vi "HB_ThreadPool.MainDIMEventListenerTask.vi"() -> ()   [LabVIEW 2009, in "HB_DIM_Examples.lvlib"]
doc: "Simple application to test the HGF_ThreadPool with a simple class."
uses:
  HB_DIM_Examples.lvlib
  HB_Factory/HB_Factory.lvclass
  lib.lib/HGF_LVC/HGF_BaseClasses/HGF_Factory/HGF_Factory.lvclass
  lib.lib/HGF_LVC/HGF_BaseClasses/HGF_Event/HGF_Event.lvclass
  lib.lib/HGF_LVC/HGF_BaseClasses/HGF_ThreadTask/HGF_ThreadTask.lvclass
  HB_Simple/HB_Simple.lvclass
  lib.lib/HGF_LVC/HGF_BaseClasses/HGF_NetworkVisitor/HGF_NetworkVisitor.lvclass
  lib.lib/HGF_LVC/HGF_BaseClasses/HGF_TriggeredEvent/HGF_TriggeredEvent.lvclass
  lib.lib/HGF_LVC/HGF_BaseClasses/HGF_PVSubscriber/HGF_PVSubscriber.lvclass
  lib.lib/HGF_LVC/HGF_DIM/HGF_DIMFactory/HGF_DIMFactory.lvclass/HGF_DIMFactory.lvclass
  lib.lib/HGF_LVC/HGF_ObjectManager/HGF_OMFactory/HGF_OMFactory.lvclass
  lib.lib/HGF_LVC/HGF_DIM/HGF_DIMDataConverter/HGF_DIMDataConverter.lvclass
  lib.lib/HGF_LVC/HGF_DIM/HGF_DIMService/HGF_DIMService.lvclass
  lib.lib/HGF_LVC/HGF_BaseClasses/HGF_ThreadPool/HGF_ThreadPool.lvclass
  lib.lib/HGF_LVC/HGF_BaseClasses/HGF_Reference/HGF_Reference.lvclass
  lib.lib/HGF_LVC/HGF_Auxiliary/HGF_Auxiliary.lvlib
  lib.lib/HGF_LVC/HGF_ObjectManager/HGF_ObjectManager.lvlib
  lib.lib/HGF_LVC/HGF_BaseClasses/HGF_Visitor/HGF_Visitor.lvclass
  lib.lib/HGF_LVC/HGF_BaseClasses/HGF_NetworkEvent/HGF_NetworkEvent.lvclass/HGF_NetworkEvent.lvclass
  lib.lib/HGF_LVC/HGF_DIM/HGF_DIMCommand/HGF_DIMCommand.lvclass
  lib.lib/DimLVEvent/LVDimInterface/LVDimInterface.lvlib
  lib.lib/HGF_LVC/HGF_DIM/HGF_DIMSubscriber/HGF_DIMSubscriber.lvclass
  lib.lib/HGF_LVC/HGF_BaseClasses/HGF_PVBase/HGF_PVBase.lvclass
panel:
  in  "y":dbl=1.0
  in  "Increment":bool
  out "objectName":string
  in  "nofObjects":i32=10
  out "Waveform Chart":dbl(graph)
  in  "timeout in ms (-1)":i32=3000
  out "nofTasksInQueueOut":i32
  out "nofTasksWaiting":i32
  out "autoIncrementLimit":i32=-1
  out "nofThreads":i32
  out "Default Destination timed out?":bool
  out "got object?":bool
  out "error":errorcluster
  in  "stop":bool
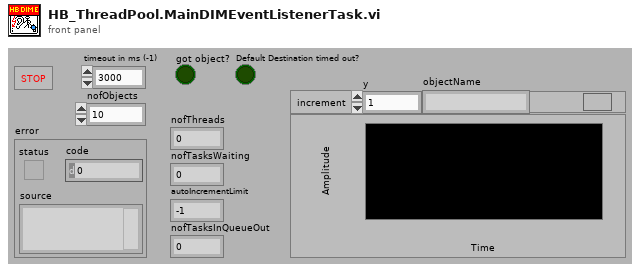
[diagram p1: front panel]
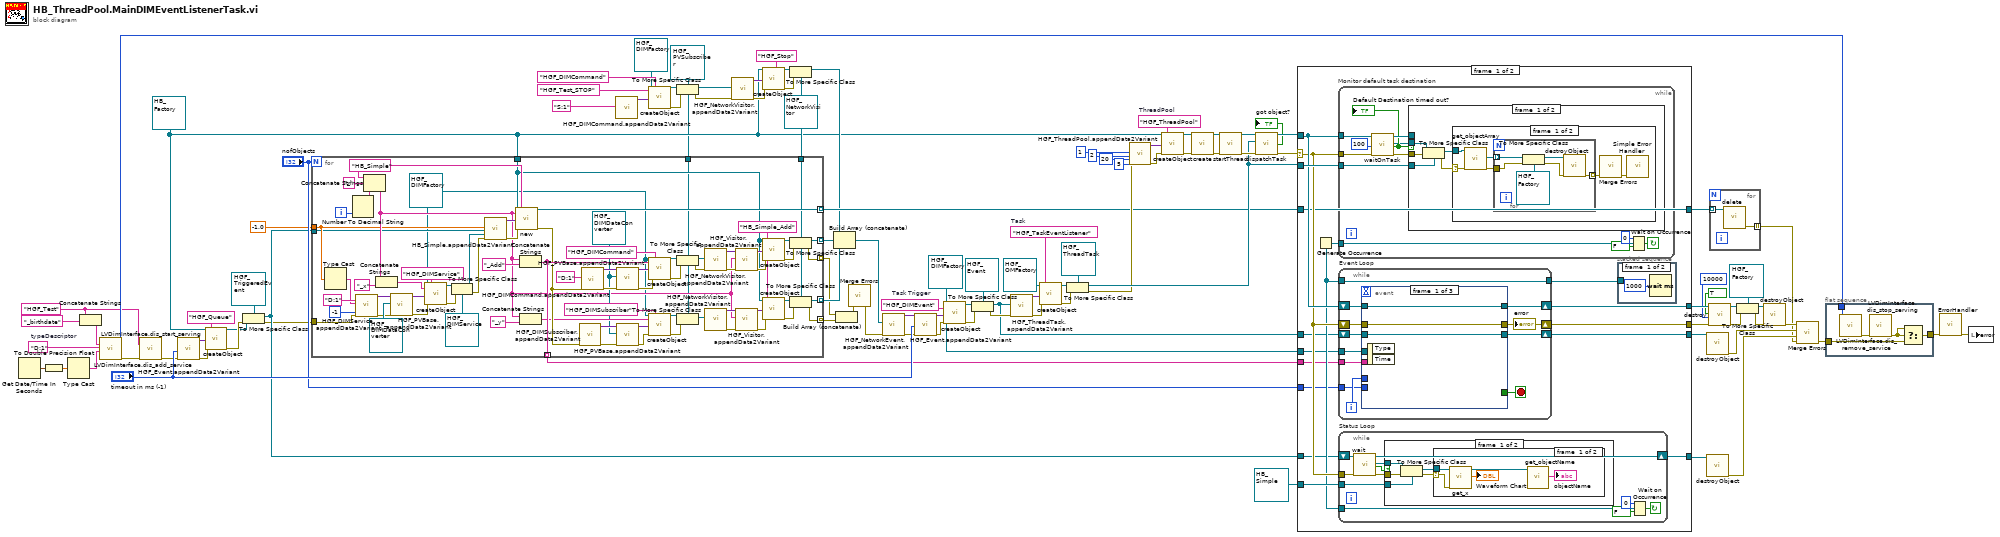
[diagram p0: block diagram]
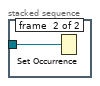
[diagram p2: hidden frame]
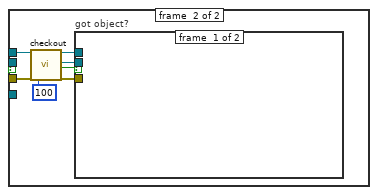
[diagram p6: hidden frame]
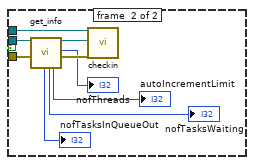
[diagram p7: hidden frame]
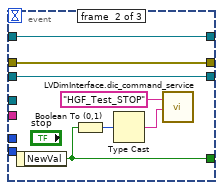
[diagram p8: hidden frame]
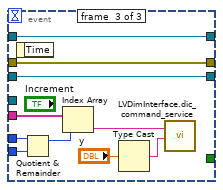
[diagram p9: hidden frame]
diagram:
  w2 = refnum<class "HGF_DIMFactory.lvclass"> refnum ("HGF_DIM.lvlib:HGF_DIMFactory.lvclass")
  w4 = refnum<class "HGF_PVSubscriber.lvclass"> refnum ("HGF_PVSubscriber")
  w7 = "HGF_Test" ("serverName")
  w13 = "D:1"  # typeDescriptor
  w35 = refnum<class "HGF_NetworkVisitor.lvclass"> refnum ("HGF_BaseClasses.lvlib:HGF_NetworkData.lvclass")
  w86 = "HGF_DIMEvent"  # Task Trigger
  w85 = "HGF_TaskEventListener"  # Task
  w78 = "HGF_ThreadPool"  # ThreadPool
  w19 = refnum<class "HB_Factory.lvclass"> refnum ("HB_Factory.lvclass")
  n1 = Get Date/Time In Seconds() -> (seconds since 1Jan1904=w10:timestamp)
  n2 = To Double Precision Float(number=w10) -> (double precision float=w11:dbl)
  n3 = Type Cast(x=w11) -> (*(type *) &x=w14:string)  [unwired: 1 out]
  n4 = Concatenate Strings(w7, "_birthdate") -> (w6:string)
  n5 = call "LVDimInterface.dis_add_service.vi"("serviceName"=w6, "typeDescriptor"=w13, "data"=w14) -> ("my_serviceID"=w9:i32, "error out"=w15:errorcluster)  [unwired: 2 in, 13 out]
  n6 = call "LVDimInterface.dis_start_serving.vi"("serverName"=w7, "error in (no error)"=w15) -> ("error out"=w12:errorcluster)  [unwired: 17 out]
  n7 = call "HGF_Event.appendData2Variant.vi"("timeout in ms (-1)"="timeout in ms (-1)", "error in (no error)"=w12) -> ("dup initData"=w64:variant, "error out"=w65:errorcluster)  [unwired: 1 in, 15 out]
  n8 = call "createObject.vi"("HGF_Factory"=w19, "initializationData"=w64, "error in (no error)"=w65, "className"="HGF_Queue") -> ("HGF_Object"=w61:refnum<class "HGF_Factory.lvclass">, "error out"=w62:errorcluster)  [unwired: 2 in, 12 out]
  n9 = To More Specific Class(target class=refnum<class "HGF_TriggeredEvent.lvclass"> refnum ("HGF_BaseClasses.lvlib:HGF_TriggeredEvent.lvclass"), reference=w61, error in=w62) -> (specific class reference=w18:refnum<class "HGF_TriggeredEvent.lvclass">, error out=w16:errorcluster)
  n10 = for {
    N: "nofObjects" -> [_]
    tunnel: [w173] -> w54 mode=indexing
    tunnel: w19 -> [w122]
    tunnel: [w163] -> w22 mode=indexing
    tunnel: [w156] -> w51 mode=indexing
    tunnel: [w162] -> w46 mode=indexing
    tunnel: w35 -> [w145]
    tunnel: [w144] -> w24 mode=indexing
    tunnel: [w143] -> w23 mode=indexing
    tunnel: w18 -> [w108]
    tunnel: -1.0 ("x") -> [w115]
    tunnel: w16 -> [w111]
    tunnel: w4 -> [w106]
    i -> [w175]
    w105 = refnum<class "HGF_DIMFactory.lvclass"> refnum ("HGF_DIM.lvlib:HGF_DIMFactory.lvclass")
    w130 = refnum<class "HGF_DIMDataConverter.lvclass"> refnum ("HGF_DIM.lvlib:HGF_DIMBaseType.lvclass")
    w146 = "HB_Simple_Add" ("className")
    w174 = "HB_Simple" ("className")
    n11 = Type Cast(x=w115) -> (*(type *) &x=w116:string)  [unwired: 1 out]
    n12 = Number To Decimal String(number=w175) -> (decimal integer string=w168:string)  [unwired: 1 out]
    n13 = call "HGF_DIMService.appendData2Variant.vi"("typeDescriptor"="D:1", "defaultData"=w116, "defaultQuality"=-1, "error in (no error)"=w111) -> ("dup initData"=w125:variant, "error out"=w126:errorcluster)  [unwired: 1 in, 13 out]
    n14 = Concatenate Strings(w174, "_" ("string"), w168) -> (w119:string)
    n15 = Concatenate Strings(w119, "_x" ("string")) -> (w118:string)
    n16 = call "HGF_PVBase.appendData2Variant.vi"("initData"=w125, "HGF_PVDataConverter"=refnum<class "HGF_DIMDataConverter.lvclass"> refnum ("HGF_DIM.lvlib:HGF_DIMBaseType.lvclass"), "error in (no error)"=w126) -> ("dup initData"=w124:variant, "error out"=w123:errorcluster)  [unwired: 15 out]
    n17 = call "createObject.vi"("HGF_Factory"=w105, "objectName"=w118, "initializationData"=w124, "error in (no error)"=w123, "className"="HGF_DIMService") -> ("HGF_Object"=w113:refnum<class "HGF_Factory.lvclass">, "error out"=w112:errorcluster)  [unwired: 1 in, 12 out]
    n18 = To More Specific Class(target class=refnum<class "HGF_DIMService.lvclass"> refnum ("HGF_DIM.lvlib:HGF_DIMService.lvclass"), reference=w113, error in=w112) -> (specific class reference=w107:refnum<class "HGF_DIMService.lvclass">, error out=w110:errorcluster)
    n19 = call "HB_Simple.appendData2Variant.vi"("x"=w115, "statusEvent"=w108, "publish_X"=w107, "error in (no error)"=w110) -> ("dup initData"=w129:variant, "error out"=w128:errorcluster)  [unwired: 1 in, 13 out]
    n20 = call "new.vi"("HGF_Factory"=w122, "objectName"=w119, "initializationData"=w129, "error in (no error)"=w128, "className"=w174) -> ("objectRef"=w173:refnum<class "HGF_Reference.lvclass">, "error out"=w141:errorcluster)  [unwired: 4 in, 9 out]
    n21 = Concatenate Strings(w119, "_Add" ("string")) -> (w156:string)
    n22 = Concatenate Strings(w119, "_y" ("string")) -> (w140:string)
    n23 = call "HGF_DIMSubscriber.appendData2Variant.vi"("error in (no error)"=w141) -> ("dup initData"=w132:variant, "error out"=w131:errorcluster)  [unwired: 4 in, 13 out]
    n24 = call "HGF_DIMCommand.appendData2Variant.vi"("typeDescriptor"="D:1", "error in (no error)"=w141) -> ("dup initData"=w137:variant, "error out"=w138:errorcluster)  [unwired: 1 in, 15 out]
    n25 = call "HGF_PVBase.appendData2Variant.vi"("initData"=w137, "HGF_PVDataConverter"=w130, "error in (no error)"=w138) -> ("dup initData"=w136:variant, "error out"=w135:errorcluster)  [unwired: 15 out]
    n26 = call "HGF_PVBase.appendData2Variant.vi"("initData"=w132, "HGF_PVDataConverter"=w130, "error in (no error)"=w131) -> ("dup initData"=w134:variant, "error out"=w133:errorcluster)  [unwired: 15 out]
    n27 = call "createObject.vi"("HGF_Factory"=w105, "objectName"=w156, "initializationData"=w136, "error in (no error)"=w135, "className"="HGF_DIMCommand") -> ("HGF_Object"=w172:refnum<class "HGF_Factory.lvclass">, "error out"=w171:errorcluster)  [unwired: 1 in, 12 out]
    n28 = call "createObject.vi"("HGF_Factory"=w105, "objectName"=w140, "initializationData"=w134, "error in (no error)"=w133, "className"="HGF_DIMSubscriber") -> ("HGF_Object"=w154:refnum<class "HGF_Factory.lvclass">, "error out"=w153:errorcluster)  [unwired: 1 in, 12 out]
    n29 = To More Specific Class(target class=w106, reference=w172, error in=w171) -> (specific class reference=w161:refnum<class "HGF_PVSubscriber.lvclass">, error out=w170:errorcluster)
    n30 = To More Specific Class(target class=w106, reference=w154, error in=w153) -> (specific class reference=w142:refnum<class "HGF_PVSubscriber.lvclass">)  [unwired: 1 out]
    n31 = call "HGF_NetworkVisitor.appendData2Variant.vi"("HGF_PVSubscriber"=w161, "error in (no error)"=w170) -> ("dup initData"=w158:variant, "error out"=w160:errorcluster)  [unwired: 1 in, 15 out]
    n32 = call "HGF_NetworkVisitor.appendData2Variant.vi"("HGF_PVSubscriber"=w142) -> ("dup initData"=w151:variant, "error out"=w149:errorcluster)  [unwired: 2 in, 15 out]
    n33 = call "HGF_Visitor.appendData2Variant.vi"("initData"=w158, "addressee"=w119, "error in (no error)"=w160) -> ("dup initData"=w157:variant, "error out"=w159:errorcluster)  [unwired: 1 in, 14 out]
    n34 = call "HGF_Visitor.appendData2Variant.vi"("initData"=w151, "addressee"=w119, "error in (no error)"=w149) -> ("dup initData"=w152:variant, "error out"=w150:errorcluster)  [unwired: 1 in, 14 out]
    n35 = call "createObject.vi"("HGF_Factory"=w122, "initializationData"=w157, "error in (no error)"=w159, "className"=w146) -> ("HGF_Object"=w165:refnum<class "HGF_Factory.lvclass">, "error out"=w164:errorcluster)  [unwired: 2 in, 12 out]
    n36 = call "createObject.vi"("HGF_Factory"=w122, "initializationData"=w152, "error in (no error)"=w150, "className"=w146) -> ("HGF_Object"=w147:refnum<class "HGF_Factory.lvclass">, "error out"=w148:errorcluster)  [unwired: 2 in, 12 out]
    n37 = To More Specific Class(target class=w145, reference=w165, error in=w164) -> (specific class reference=w162:refnum<class "HGF_NetworkVisitor.lvclass">, error out=w163:errorcluster)
    n38 = To More Specific Class(target class=w145, reference=w147, error in=w148) -> (specific class reference=w144:refnum<class "HGF_NetworkVisitor.lvclass">, error out=w143:errorcluster)
  }
  n39 = call "HGF_DIMCommand.appendData2Variant.vi"("typeDescriptor"="S:1") -> ("dup initData"=w41:variant)  [unwired: 2 in, 16 out]
  n40 = call "createObject.vi"("HGF_Factory"=refnum<class "HGF_DIMFactory.lvclass"> refnum ("HGF_DIM.lvlib:HGF_DIMFactory.lvclass"), "objectName"="HGF_Test_STOP", "initializationData"=w41, "className"="HGF_DIMCommand") -> ("HGF_Object"=w37:refnum<class "HGF_Factory.lvclass">, "error out"=w38:errorcluster)  [unwired: 2 in, 12 out]
  n41 = To More Specific Class(target class=w4, reference=w37, error in=w38) -> (specific class reference=w45:refnum<class "HGF_PVSubscriber.lvclass">, error out=w39:errorcluster)
  n42 = call "HGF_NetworkVisitor.appendData2Variant.vi"("HGF_PVSubscriber"=w45, "error in (no error)"=w39) -> ("dup initData"=w32:variant, "error out"=w31:errorcluster)  [unwired: 1 in, 15 out]
  n43 = call "createObject.vi"("HGF_Factory"=w19, "initializationData"=w32, "error in (no error)"=w31, "className"="HGF_Stop") -> ("HGF_Object"=w43:refnum<class "HGF_Factory.lvclass">, "error out"=w44:errorcluster)  [unwired: 2 in, 12 out]
  n44 = To More Specific Class(target class=w35, reference=w43, error in=w44) -> (specific class reference=w33:refnum<class "HGF_NetworkVisitor.lvclass">)  [unwired: 1 out]
  n45 = Build Array (concatenate)(w33, w46, w24) -> (w47:refnum<class "HGF_NetworkVisitor.lvclass">[])
  n46 = Build Array (concatenate)(w22, w23) -> (w21:errorcluster[])
  n47 = call <vilib>:"Merge Errors.vi"("error array in"=w21) -> ("error out"=w48:errorcluster)  [unwired: 3 in, 3 out]
  n48 = call "HGF_NetworkEvent.appendData2Variant.vi"("callbackVisitors"=w47, "error in (no error)"=w48) -> ("dup initData"=w50:variant, "error out"=w49:errorcluster)  [unwired: 1 in, 15 out]
  n49 = call "HGF_Event.appendData2Variant.vi"("initData"=w50, "timeout in ms (-1)"="timeout in ms (-1)", "error in (no error)"=w49) -> ("dup initData"=w91:variant, "error out"=w90:errorcluster)  [unwired: 1 in, 14 out]
  n50 = call "createObject.vi"("HGF_Factory"=w2, "initializationData"=w91, "error in (no error)"=w90, "className"=w86) -> ("HGF_Object"=w83:refnum<class "HGF_Factory.lvclass">, "error out"=w92:errorcluster)  [unwired: 2 in, 12 out]
  n51 = To More Specific Class(target class=refnum<class "HGF_Event.lvclass"> refnum ("HGF_BaseClasses.lvlib:HGF_Event.lvclass"), reference=w83, error in=w92) -> (specific class reference=w67:refnum<class "HGF_Event.lvclass">, error out=w77:errorcluster)
  n52 = call "HGF_ThreadTask.appendData2Variant.vi"("taskTrigger"=w67, "error in (no error)"=w77) -> ("dup initData"=w76:variant, "error out"=w75:errorcluster)  [unwired: 4 in, 12 out]
  n53 = call "createObject.vi"("HGF_Factory"=refnum<class "HGF_OMFactory.lvclass"> refnum ("HGF_ObjectManager.lvlib:HGF_OMFactory.lvclass"), "initializationData"=w76, "error in (no error)"=w75, "className"=w85) -> ("HGF_Object"=w82:refnum<class "HGF_Factory.lvclass">, "error out"=w89:errorcluster)  [unwired: 2 in, 12 out]
  n54 = To More Specific Class(target class=refnum<class "HGF_ThreadTask.lvclass"> refnum ("HGF_BaseClasses.lvlib:HGF_ThreadTask.lvclass"), reference=w82, error in=w89) -> (specific class reference=w68:refnum<class "HGF_ThreadTask.lvclass">, error out=w58:errorcluster)
  n55 = call "HGF_ThreadPool.appendData2Variant.vi"("initialNofThreads (0)"=1 ("initialNofThreads"), "incThreads(1)"=2 ("incThreads"), "maxNofThreads (-1:unlimited)"=20 ("maxNofThreads"), "error in (no error)"=w58, "autoIncrementLimit (-1)"=5) -> ("dup initData"=w103:variant, "error out"=w59:errorcluster)  [unwired: 2 in, 11 out]
  n56 = call "createObject.vi"("HGF_Factory"=w19, "initializationData"=w103, "error in (no error)"=w59, "className"=w78) -> ("HGF_Object"=w84:refnum<class "HGF_Factory.lvclass">, "error out"=w102:errorcluster)  [unwired: 2 in, 12 out]
  n57 = call "create.vi"("Object"=w84, "error in (no error)"=w102) -> ("HGF_Reference"=w104:refnum<class "HGF_Reference.lvclass">, "error out"=w98:errorcluster)  [unwired: 1 in, 15 out]
  n58 = call "startThread.vi"("HGF_ThreadPool_Reference"=w104, "error in (no error)"=w98) -> ("dup HGF_ThreadPool_Reference"=w73:refnum<class "HGF_Reference.lvclass">, "error out"=w71:errorcluster)  [unwired: 1 in, 15 out]
  n59 = call "dispatchTask.vi"("HGF_ThreadPool_Reference"=w73, "HGF_ThreadTask"=w68, "error in (no error)"=w71) -> ("dup HGF_ThreadPool_Reference"=w72:refnum<class "HGF_Reference.lvclass">, "got object?"=→"got object?":bool, "error out"=w70:errorcluster)  [unwired: 1 in, 13 out]
  n60 = case shown="No Error" w70 {
    selector: w70 -> [w187 w296]
    tunnel: w72 -> [w189 w297]
    tunnel: [w192 w297] -> w88
    tunnel: w68 -> [w190 _]
    tunnel: [w191 w296] -> w87
    tunnel: w67 -> [w182 w294]
    tunnel: w18 -> [w183 w295]
    tunnel: refnum<class "HB_Simple.lvclass"> refnum ("HGF_BaseClass_Examples.lvlib:HB_Simple.lvclass") -> [w186 _]
    tunnel: w2 -> [w184 _]
    tunnel: [w181 w295] -> w56
    tunnel: [w180 w294] -> w55
    tunnel: w54 -> [w179 w293]
    tunnel: [w179 w293] -> w53
    tunnel: "nofObjects" -> [w178 _]
    tunnel: w51 -> [w177 _]
    frame #0 {
      n61 = Generate Occurrence() -> (w185:refnum<k4>)
      n62 = while "Monitor default task destination" {
        tunnel: w190 -> [w223]
        tunnel: w189 -> [w222]
        tunnel: w187 -> [w221]
        tunnel: w185 -> [w216]
        stop <- w217 continue-if-true
        n63 = call "waitOnTask.vi"("HGF_ThreadPool_Reference"=w222, "timeout in ms (-1)"=100, "error in (no error)"=w221) -> ("dup HGF_ThreadPool_Reference"=w227:refnum<class "HGF_Reference.lvclass">, "HGF_Task"=w225:refnum<class "HGF_ThreadTask.lvclass">, "timed out?"=w226:bool, "error out"=w220:errorcluster)  [unwired: 13 out]
        "Default Destination timed out?" <- w226
        n64 = case "timed out?" shown="True" w226 {
          tunnel: w225 -> [w232 _]
          tunnel: w220 -> [w231 w245]
          tunnel: w227 -> [_ w246]
          tunnel: w223 -> [w228 _]
          frame #0 {
            n65 = To More Specific Class(target class=w228, reference=w232, error in=w231) -> (specific class reference=w230:refnum<class "HGF_ThreadTask.lvclass">, error out=w229:errorcluster)
            n66 = case shown="No Error" w229 {
              selector: w229 -> [w237 _]
              tunnel: w230 -> [w238 _]
              frame #0 {
                n67 = call "get_objectArray.vi"("HGF_ThreadTask"=w238, "error in (no error)"=w237) -> ("objectArray"=w233:refnum<class>[], "error out"=w235:errorcluster)  [unwired: 16 out]
                n68 = for {
                  tunnel: w235 -> [w241]
                  tunnel: [w244] -> w236 mode=indexing
                  tunnel: w233 -> [w243] mode=indexing
                  n69 = To More Specific Class(target class=refnum<class "HGF_Factory.lvclass"> refnum ("HGF_BaseClasses.lvlib:HGF_Factory.lvclass"), reference=w243, error in=w241) -> (specific class reference=w242:refnum<class "HGF_Factory.lvclass">, error out=w240:errorcluster)
                  n70 = call "destroyObject.vi"("HGF_Factory"=w242, "error in (no error)"=w240) -> ("error out"=w244:errorcluster)  [unwired: 17 out]
                }
                n71 = call <vilib>:"Merge Errors.vi"("error array in"=w236) -> ("error out"=w234:errorcluster)  [unwired: 3 in, 3 out]
                n72 = call <vilib>:"Simple Error Handler.vi"("error in (no error)"=w234) -> ()  [unwired: 1 in, 8 out]
              }
              frame #1 {
              }
            }
          }
          frame #1 {
            n73 = call "checkout.vi"("HGF_ThreadPool_Reference"=w246, "timeout in ms (-1)"=100, "error in (no error)"=w245) -> ("dup HGF_ThreadPool_Reference"=w247:refnum<class "HGF_Reference.lvclass">, "HGF_ThreadPool"=w248:refnum<class "HGF_ThreadPool.lvclass">, "got object?"=w251:bool, "error out"=w249:errorcluster)  [unwired: 13 out]
            n74 = case "got object?" shown="True" w251 {
              tunnel: w247 -> [_ w260]
              tunnel: w248 -> [_ w259]
              tunnel: w249 -> [_ w258]
              frame #0 {
              }
              frame #1 {
                n75 = call "get_info.vi"("HGF_ThreadPool"=w259, "error in (no error)"=w258) -> ("nofTasksInQueueOut"=→"nofTasksInQueueOut":i32, "nofTasksWaiting"=→"nofTasksWaiting":i32, "autoIncrementLimit"=→"autoIncrementLimit":i32, "dup HGF_ThreadPool"=w256:refnum<class "HGF_ThreadPool.lvclass">, "nofThreads"=→"nofThreads":i32, "error out"=w257:errorcluster)  [unwired: 12 out]
                n76 = call "checkin.vi"("HGF_Reference"=w260, "Object"=w256, "error in (no error)"=w257) -> ()  [unwired: 1 in, 16 out]
              }
            }
          }
        }
        n77 = Wait on Occurrence(1:FALSE ("ignore previous (T)"), 2:w216, 3:0 ("ms timeout (-1)")) -> (0:w217:bool)
      }
      n78 = while "Event Loop" {
        shift-right: [w271] -> w192
        shift-left: w189 -> [w270]
        shift-right: [w261] -> w191
        shift-left: w187 -> [w272]
        tunnel: w185 -> [w267]
        tunnel: [w267] -> w188
        tunnel: w184 -> [w268]
        shift-right: [w265] -> w180
        shift-left: w182 -> [w269]
        tunnel: w178 -> [w263]
        tunnel: w177 -> [w262]
        i -> [w264]
        stop <- w266 stop-if-true
        n79 = event shown="[2] \"Increment\": Value Change" {
          selector: _ -> [_ _ _]
          dyn-events: _ -> [_ _ _]
          timeout: _ -> [_ _ _]
          tunnel: [_ w278 _] -> w266
          tunnel: [w274 w280 w287] -> w261
          tunnel: w272 -> [w274 w280 w287]
          tunnel: [w275 w282 w292] -> w271
          tunnel: w270 -> [w275 w282 w292]
          tunnel: w269 -> [w273 w281 w286]
          tunnel: w268 -> [_ _ _]
          tunnel: [w273 w281 w286] -> w265
          tunnel: w264 -> [_ _ w291]
          tunnel: w263 -> [_ _ w290]
          tunnel: w262 -> [_ _ w289]
          event #0 {
            n80 = event-data() -> ()  [unwired: 3 out]
          }
          event #1 {
            n81 = event-data() -> ("NewVal"=w278:bool)  [unwired: 1 out]
            n82 = Boolean To (0,1)(Boolean=w278) -> (0, 1=w276:i16)
            n83 = Type Cast(x=w276) -> (*(type *) &x=w277:string)  [unwired: 1 out]
            n84 = call "LVDimInterface.dic_command_service.vi"("commandName"="HGF_Test_STOP" ("objectName"), "data"=w277) -> ()  [unwired: 1 in, 17 out]
          }
          event #2 {
            n85 = event-data() -> ()  [unwired: 2 out]
            n86 = Quotient & Remainder(x=w291, y=w290) -> (x-y*floor(x/y)=w288:i32)  [unwired: 1 out]
            n87 = Index Array(array=w289, index=w288) -> (element=w285:string)
            n88 = Type Cast(x="y") -> (*(type *) &x=w284:string)  [unwired: 1 out]
            n89 = call "LVDimInterface.dic_command_service.vi"("commandName"=w285, "data"=w284) -> ()  [unwired: 1 in, 17 out]
          }
        }
        "error" <- w261
      }
      n90 = while "Status Loop" {
        tunnel: w187 -> [w204]
        tunnel: w186 -> [w201]
        tunnel: w185 -> [w196]
        shift-right: [w195] -> w181
        shift-left: w183 -> [w205]
        stop <- w197 continue-if-true
        n91 = call-dynamic "wait.vi"("HGF_Event"=w205, "error in (no error)"=w204) -> ("dup HGF_Event"=w195:refnum<class "HGF_TriggeredEvent.lvclass">, "Object"=w202:refnum<class>, "timed out"=w200:bool, "error out"=w203:errorcluster)  [unwired: 2 in, 12 out]
        n92 = case shown="False" w200 {
          tunnel: w203 -> [w210 _]
          tunnel: w202 -> [w209 _]
          tunnel: w201 -> [w208 _]
          frame #0 {
            n93 = To More Specific Class(target class=w208, reference=w209, error in=w210) -> (specific class reference=w206:refnum<class "HB_Simple.lvclass">, error out=w207:errorcluster)
            n94 = case shown="No Error" w207 {
              selector: w207 -> [w214 _]
              tunnel: w206 -> [w215 _]
              frame #0 {
                n95 = call "get_x.vi"("HB_Simple"=w215, "error in (no error)"=w214) -> ("dup HB_Simple"=w212:refnum<class "HB_Simple.lvclass">, "x"=→"Waveform Chart":dbl)  [unwired: 16 out]
                n96 = call "get_objectName.vi"("HGF_Factory"=w212) -> ("objectName"=→"objectName":string)  [unwired: 1 in, 17 out]
              }
              frame #1 {
              }
            }
          }
          frame #1 {
          }
        }
        n97 = Wait on Occurrence(1:FALSE ("ignore previous (T)"), 2:w196, 3:0 ("ms timeout (-1)")) -> (0:w197:bool)
      }
      n98 = stacked-sequence {
        tunnel: w188 -> [_ w194]
        frame #0 {
          n99 = Wait (ms)(milliseconds to wait=u32 1000) -> ()  [unwired: 1 out]
        }
        frame #1 {
          n100 = Set Occurrence(w194) -> ()
        }
      }
    }
    frame #1 {
    }
  }
  n101 = call "destroyObject.vi"("HGF_Factory"=w55) -> ("error out"=w29:errorcluster)  [unwired: 1 in, 17 out]
  n102 = call "destroyObject.vi"("HGF_Factory"=w56) -> ("error out"=w28:errorcluster)  [unwired: 1 in, 17 out]
  n103 = call "destroy.vi"("HGF_Reference"=w88, "wait for activity? (F)"=TRUE, "timeout /ms (-1)"=10000, "error in (no error)"=w87) -> ("Object"=w97:refnum<class>, "error out"=w95:errorcluster)  [unwired: 14 out]
  n104 = for {
    tunnel: w53 -> [w299] mode=indexing
    tunnel: [w298] -> w27 mode=indexing
    n105 = call "delete.vi"("objectRef"=w299) -> ("error out"=w298:errorcluster)  [unwired: 3 in, 3 out]
  }
  n106 = To More Specific Class(target class=refnum<class "HGF_Factory.lvclass"> refnum ("HGF_BaseClasses.lvlib:HGF_Factory.lvclass"), reference=w97, error in=w95) -> (specific class reference=w96:refnum<class "HGF_Factory.lvclass">, error out=w94:errorcluster)
  n107 = call "destroyObject.vi"("HGF_Factory"=w96, "error in (no error)"=w94) -> ("error out"=w30:errorcluster)  [unwired: 17 out]
  n108 = call <vilib>:"Merge Errors.vi"("error array in"=w27, "error in 3 (no error)"=w28, "error in 2 (no error)"=w29, "error in 1 (no error)"=w30) -> ("error out"=w26:errorcluster)  [unwired: 3 out]
  n109 = flat-sequence {
    tunnel: w26 -> [w303]
    tunnel: [w302] -> w25
    tunnel: w9 -> [w300]
    frame #0 {
      n110 = call "LVDimInterface.dis_remove_service.vi"("my_serviceID"=w300) -> ("error out"=w301:errorcluster)  [unwired: 2 in, 16 out]
      n111 = call "LVDimInterface.dis_stop_serving.vi"("error in (no error)"=w301) -> ("error out"=w304:errorcluster)  [unwired: 18 out]
      n112 = Select(t=w304, s=w304, f=w303) -> (s? t:f=w302:errorcluster)
    }
  }
  n113 = call "ErrorHandler.vi"("error in (no error)"=w25) -> ("error out"=w5:errorcluster)  [unwired: 6 in, 12 out]
  n114 = local write "error"(w5) -> ()
